vi "TagBus_Factory.vi"(10 "TagDescriptions":refnum<class "tag descriptor.lvclass">[](array[class])=[refnum, refnum, refnum, refnum]) -> (3 "TagBus DVR":refnum<data-value>)   [LabVIEW 2015, in "TagBus.lvclass"]
uses:
  TagBus.lvclass
  <vilib>/NI/Tag Bus/tag/tag descriptor.lvclass
  <vilib>/NI/Tag Bus/dictionary/data dictionary.lvclass/data dictionary.ctl
  TagBus.lvclass/TagBus.ctl
  <vilib>/NI/Tag Bus/dictionary/data dictionary.lvclass
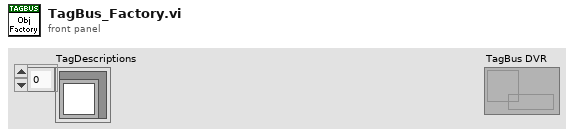
[diagram p1: front panel]
types:
  T1 = typedef "tag bus.lvlib/data table.lvlib/data table.ctl" = cluster{"Double":dbl[], "Single":sgl[], "I64":i64[], "I32":i32[], "I16":i16[], "I8":i8[], "U64":u64[], "U32":u32[], "U16":u16[], "U8":u8[], "Boolean":bool[], "String":string[], "Array of Double":cluster{"DBL Array":dbl[]}[], "Array of Single":cluster{"SGL Array":sgl[]}[], "Array of I64":cluster{"I64 Array":i64[]}[], "Array of I32":cluster{"I32 Array":i32[]}[], "Array of I16":cluster{"I16 Array":i16[]}[], "Array of I8":cluster{"I8 Array":i8[]}[], "Array of U64":cluster{"U64 Array":u64[]}[], "Array of U32":cluster{"U32 Array":u32[]}[], "Array of U16":cluster{"U16 Array":u16[]}[], "Array of U8":cluster{"U8 Array":u8[]}[], "Array of Boolean":cluster{"Boolean Array":bool[]}[], "Array of String":cluster{"String Array":string[]}[]}
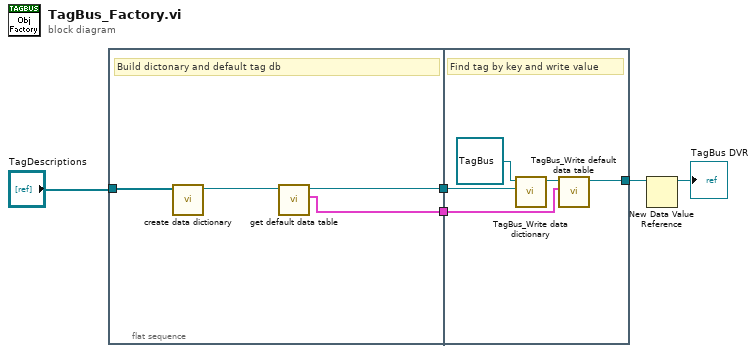
[diagram p0: block diagram]
diagram:
  n1 = flat-sequence {
    tunnel: [w8] -> w5
    tunnel: [w7] -> w4
    tunnel: "TagDescriptions" -> [w6]
    tunnel: w5 -> [w11]
    tunnel: w4 -> [w12]
    tunnel: [w10] -> w2
    frame #0 {
      # "Build dictonary and default tag db"
      n2 = call <vilib>:"create data dictionary.vi"("system tags"=w6) -> ("data dictionary"=w9:refnum<class "data dictionary.lvclass">)  [unwired: 9 in, 1 out]
      n3 = call <vilib>:"get default data table.vi"("data dictionary in"=w9) -> ("default data table"=w8:T1, "data dictionary out"=w7:refnum<class "data dictionary.lvclass">)  [unwired: 9 in]
    }
    frame #1 {
      # "Find tag by key and write value"
      n4 = call "TagBus_Write data dictionary.vi"("tag bus:data dictionary"=w12, "TagBus in"=refnum<class "TagBus.lvclass"> refnum ("TagBus.lvclass")) -> ("TagBus out"=w13:refnum<class "TagBus.lvclass">)  [unwired: 9 in]
      n5 = call "TagBus_Write default data table.vi"("data table"=w11, "TagBus in"=w13) -> ("TagBus out"=w10:refnum<class "TagBus.lvclass">)  [unwired: 9 in]
    }
  }
  n6 = New Data Value Reference(data value=w2) -> (data value reference=→"TagBus DVR":refnum<data-value>)  [unwired: 1 in, 1 out]
